vi "GetChannelCoupling.vi"(8 "error in (no error)":errorcluster, 11 "TektronixDPO_PhysicalDevice.lvclass":refnum<class "TektronixDPO_PhysicalDevice.lvclass">) -> (0 "error out":errorcluster, 3 "TektronixDPO_PhysicalDevice.lvclassOut":refnum<class "TektronixDPO_PhysicalDevice.lvclass">)   [LabVIEW 2013, in "TektronixDPO_PhysicalDevice.lvclass"]
doc: "Read from the phsyical device the offset relative to the specified channel"
uses:
  TektronixDPO_PhysicalDevice.lvclass
  shared/Typdefs/Choice11.ctl
  TektronixDPO_PhysicalDevice.lvclass/TektronixDPO_PhysicalDevice.ctl
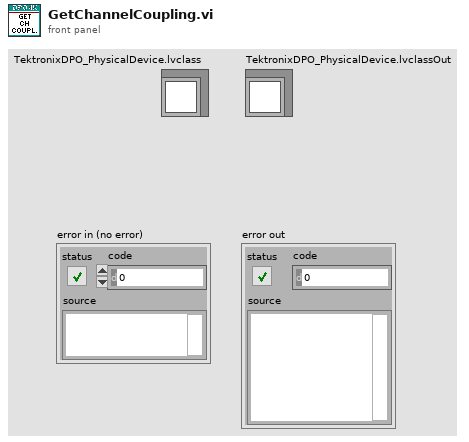
[diagram p1: front panel]
types:
  T1 = typedef "Choice11.ctl" = enum16{"AC", "DC", "Ground"}
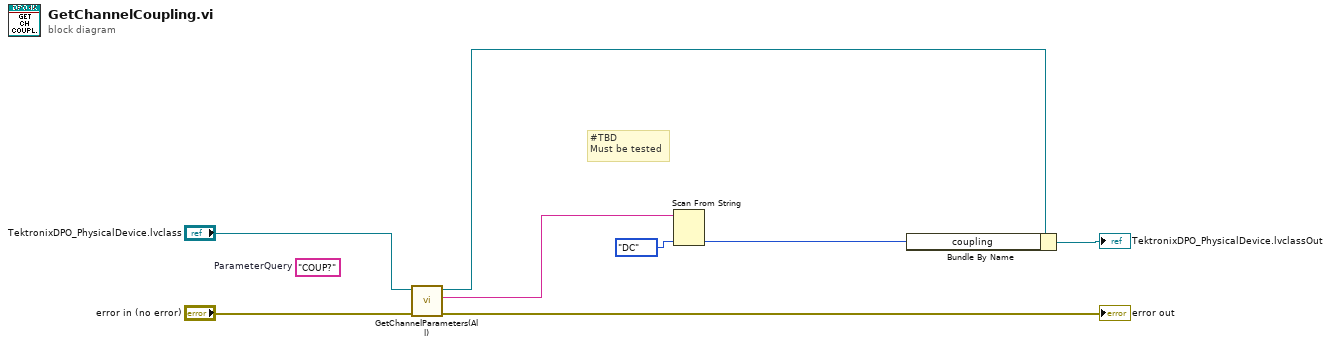
[diagram p0: block diagram]
diagram:
  (unwired) "COUP?"  # ParameterQuery
  # "#TBD\nMust be tested"
  n1 = call "GetChannelParameters(All).vi"("error in (no error)"="error in (no error)", "TektronixDPO_PhysicalDevice in"="TektronixDPO_PhysicalDevice.lvclass") -> ("error out"=→"error out":errorcluster, "Response"=w3:string, "TektronixDPO_PhysicalDevice out"=w4:refnum<class "TektronixDPO_PhysicalDevice.lvclass">)  [unwired: 7 in]
  n2 = Scan From String(input string=w3, default 1=Choice11."DC" ("Channel0")) -> (output 1=w1:T1)  [unwired: 3 in, 3 out]
  n3 = Bundle By Name(cluster=w4, "coupling"=w1) -> (→"TektronixDPO_PhysicalDevice.lvclassOut":refnum<class "TektronixDPO_PhysicalDevice.lvclass">)
